vi "Library_AttitudeControl_init.vi"(8 "error in (no error)":errorcluster) -> (0 "error out":errorcluster)   [LabVIEW 2013]
uses:
  My Computer/Controls/Steering Inputs.ctl
  My Computer/Controls/Attitude Controllers Parameters.ctl
  My Computer/Controls/EKF_Settings.ctl
  My Computer/Controls/Intuitive Steering.ctl
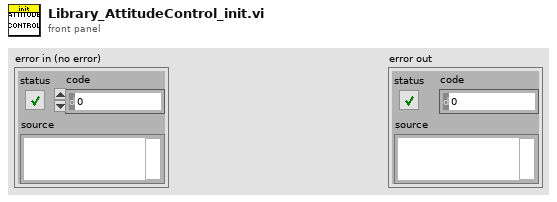
[diagram p1: front panel]
types:
  T1 = typedef "Intuitive Steering.ctl" = cluster{"Frequency (Hz):":dbl, "Max. Amplitude (°):":dbl, "Phase Shift (/Pi):":dbl, "Flap (°):":dbl, "Flap Saturation:":dbl}
  T2 = typedef "EKF_Settings.ctl" = cluster{"Gravity constant":dbl, "Filter Version":enum16{"IMU Only", "IMU & Pressure", "IMU, Pressure, Compass"}, "Initial Biases":cluster{"Gyro_Bias_nit_x":dbl, "Gyro_Bias_init_y":dbl, "Gyro_Bias_init_z":dbl, "Acc_Bias_init_x":dbl, "Acc_Bias_init_y":dbl, "Acc_Bias_init_z":dbl}, "Use Compass on initialisation":bool, "Initial Biases Covariances":cluster{"Initial_covariance_Gyro_Bias":dbl, "Initial_covariance_Acc_Bias":dbl}, "Magnetic-Field-Vector [utesla]":cluster{"Magf_N_x":dbl, "Magf_N_y":dbl, "Magf_N_z":dbl}, "IMU_Sigmas":cluster{"Sigma_w":dbl, "Sigma_wb":dbl, "Sigma_a":dbl, "Sigma_ab":dbl, "Sigma_m":dbl}, "Measurement Sigmas":cluster{"Sigma_v":dbl, "Sigma_depth":dbl}}
  T3 = typedef "Attitude Controllers Parameters.ctl" = cluster{"ARW on":cluster{"Phi":bool, "Theta":bool, "Psi":bool}, "kp":cluster{"kp Phi":dbl, "kp Theta":dbl, "kp Psi":dbl}, "Ti":cluster{"Ti Phi":dbl, "Ti Theta":dbl, "Ti Psi":dbl}, "Integrator enabled range [rad      ":cluster{"I_E Phi":dbl, "I_E Theta":dbl, "I_E Psi":dbl}}
  T4 = cluster{"New attitude phi":dbl, "New attitude theta":dbl, "New attitude psi":dbl}
  T5 = typedef "Steering Inputs.ctl" = cluster{"X":dbl, "Y":dbl, "Z":dbl, "phi":dbl, "theta":dbl, "psi":dbl}
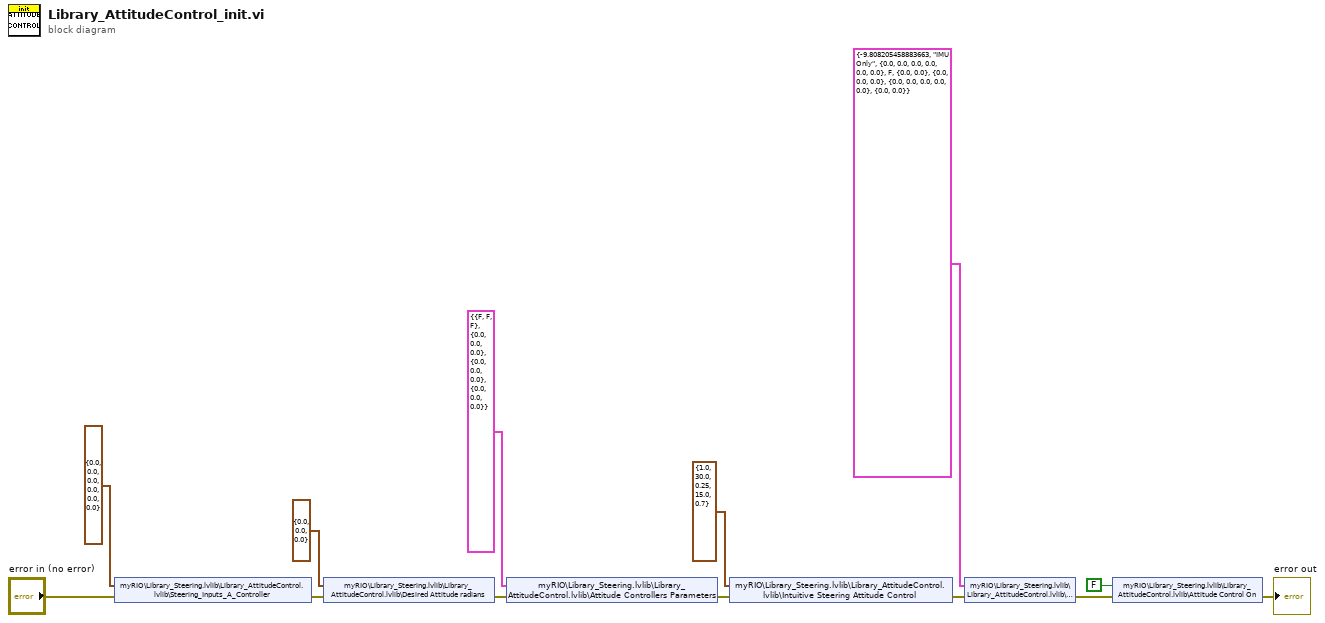
[diagram p0: block diagram]
diagram:
  n1 = shared-variable "myRIO\\Library_Steering.lvlib\\Library_AttitudeControl.lvlib\\Steering_Inputs_A_Controller"(T5 {"X"=0.0, "Y"=0.0, "Z"=0.0, "phi"=0.0, "theta"=0.0, "psi"=0.0} ("Steering_Inputs_A_Controller"), error in="error in (no error)") -> (error out=w12:errorcluster)
  n2 = shared-variable "myRIO\\Library_Steering.lvlib\\Library_AttitudeControl.lvlib\\Desired Attitude radians"(T4 {"New attitude phi"=0.0, "New attitude theta"=0.0, "New attitude psi"=0.0} ("Desired Attitude radians"), error in=w12) -> (error out=w11:errorcluster)
  n3 = shared-variable "myRIO\\Library_Steering.lvlib\\Library_AttitudeControl.lvlib\\Attitude Controllers Parameters"(T3 {"ARW on"={"Phi"=FALSE, "Theta"=FALSE, "Psi"=FALSE}, "kp"={"kp Phi"=0.0, "kp Theta"=0.0, "kp Psi"=0.0}, "Ti"={"Ti Phi"=0.0, "Ti Theta"=0.0, "Ti Psi"=0.0}, "Integrator enabled range [rad      "={"I_E Phi"=0.0, "I_E Theta"=0.0, "I_E Psi"=0.0}} ("Attitude Controllers Parameters"), error in=w11) -> (error out=w2:errorcluster)
  n4 = shared-variable "myRIO\\Library_Steering.lvlib\\Library_AttitudeControl.lvlib\\Intuitive Steering Attitude Control"(T1 {"Frequency (Hz):"=1.0, "Max. Amplitude (°):"=30.0, "Phase Shift (/Pi):"=0.25, "Flap (°):"=15.0, "Flap Saturation:"=0.7} ("Intuitive Steering Attitude Control"), error in=w2) -> (error out=w1:errorcluster)
  n5 = shared-variable "myRIO\\Library_Steering.lvlib\\Library_AttitudeControl.lvlib\\EKF_Settings"(T2 {"Gravity constant"=-9.808205458883663, "Filter Version"=enum."IMU Only", "Initial Biases"={"Gyro_Bias_nit_x"=0.0, "Gyro_Bias_init_y"=0.0, "Gyro_Bias_init_z"=0.0, "Acc_Bias_init_x"=0.0, "Acc_Bias_init_y"=0.0, "Acc_Bias_init_z"=0.0}, "Use Compass on initialisation"=FALSE, "Initial Biases Covariances"={"Initial_covariance_Gyro_Bias"=0.0, "Initial_covariance_Acc_Bias"=0.0}, "Magnetic-Field-Vector [utesla]"={"Magf_N_x"=0.0, "Magf_N_y"=0.0, "Magf_N_z"=0.0}, "IMU_Sigmas"={"Sigma_w"=0.0, "Sigma_wb"=0.0, "Sigma_a"=0.0, "Sigma_ab"=0.0, "Sigma_m"=0.0}, "Measurement Sigmas"={"Sigma_v"=0.0, "Sigma_depth"=0.0}} ("EKF_Settings"), error in=w1) -> (error out=w4:errorcluster)
  n6 = shared-variable "myRIO\\Library_Steering.lvlib\\Library_AttitudeControl.lvlib\\Attitude Control On"(FALSE ("Attitude Control On"), error in=w4) -> (error out=→"error out":errorcluster)
